vi "Manage Springboards.vi"() -> ()   [LabVIEW 2016]
panel:
  in  "Open in Explorer":bool
  in  "Open VI":bool
  in  "Delete":bool
  in  "Springboards List":i32[](listbox)
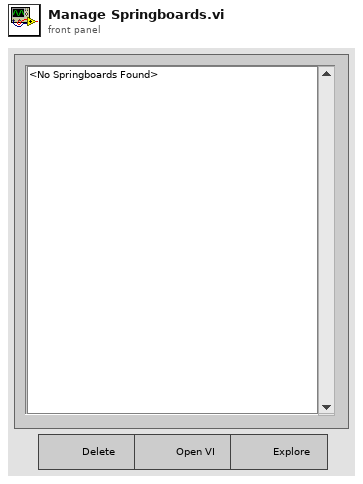
[diagram p1: front panel]
types:
  T1 = cluster{"Base Path":path, "Selected Items":i32[], "Springboard List":string[]}
  T2 = enum16{"Init", "Wait", "Delete", "Open", "Explore", "Exit"}
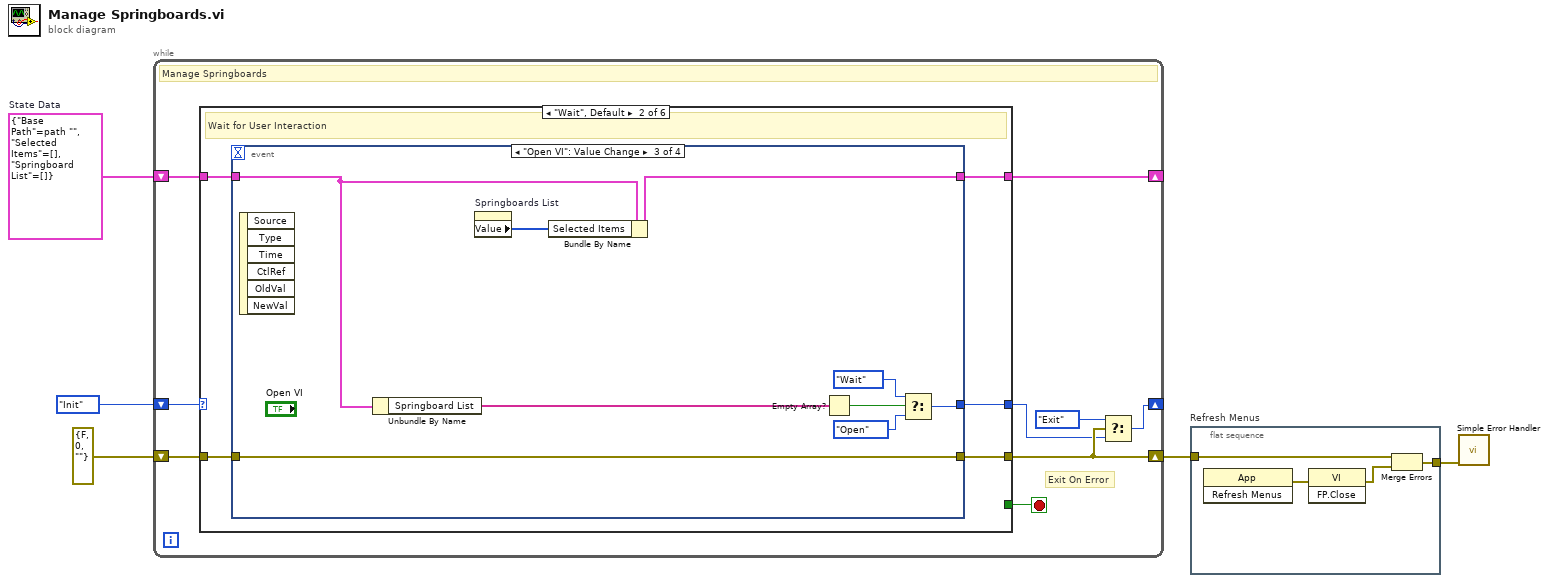
[diagram p0: block diagram]
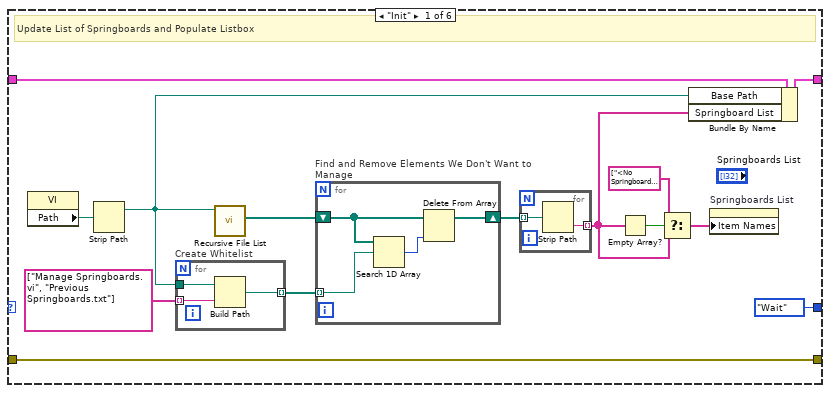
[diagram p2: hidden frame]
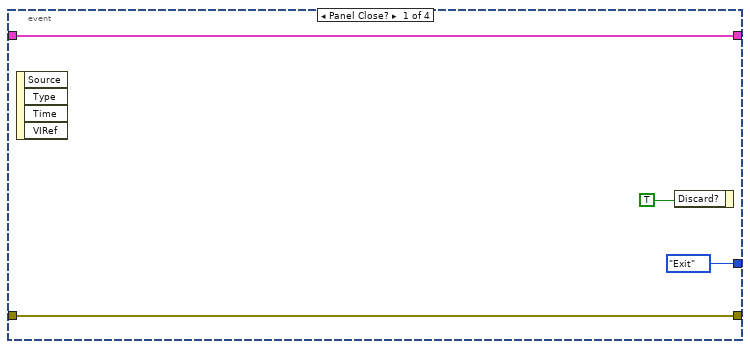
[diagram p3: hidden frame]
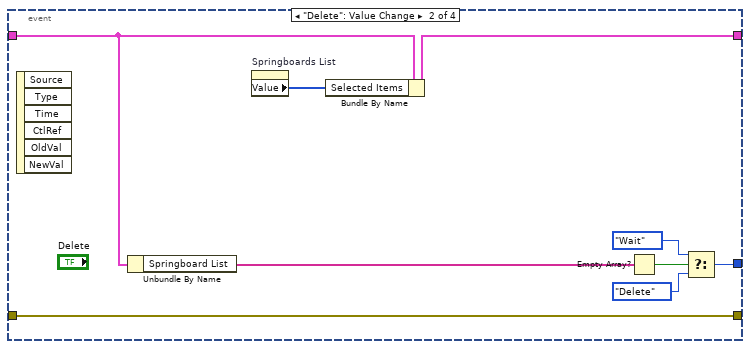
[diagram p4: hidden frame]
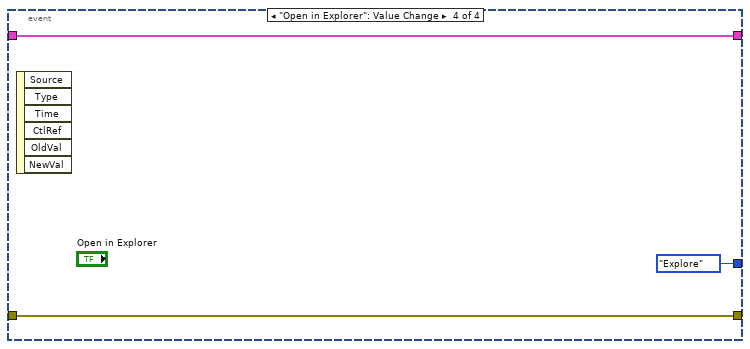
[diagram p5: hidden frame]
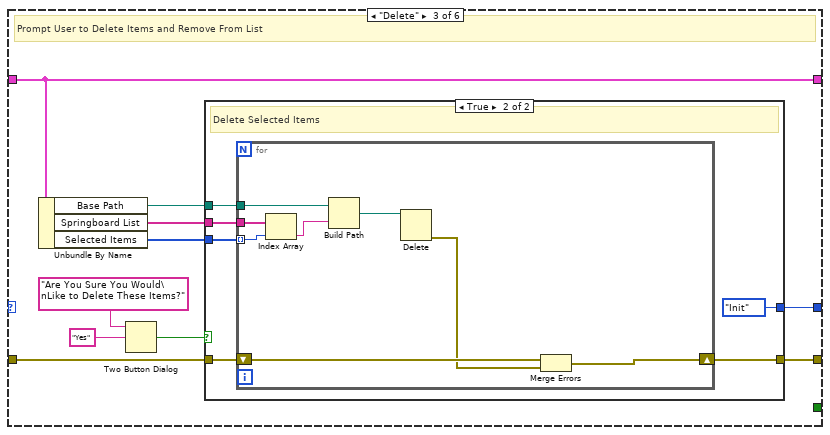
[diagram p6: hidden frame]
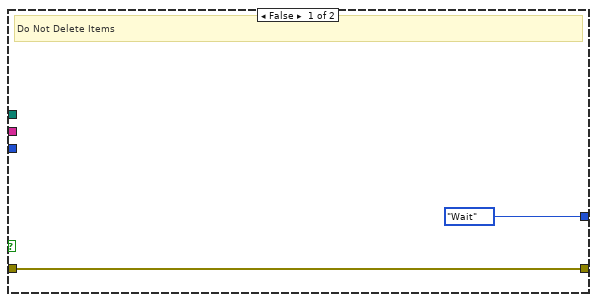
[diagram p7: hidden frame]
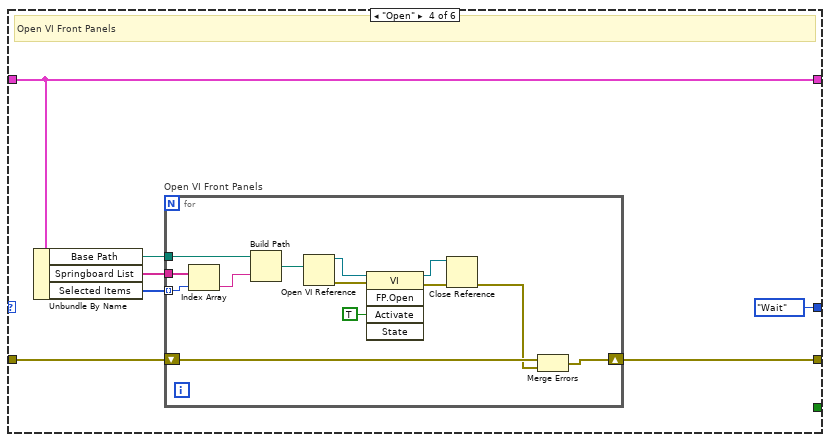
[diagram p8: hidden frame]
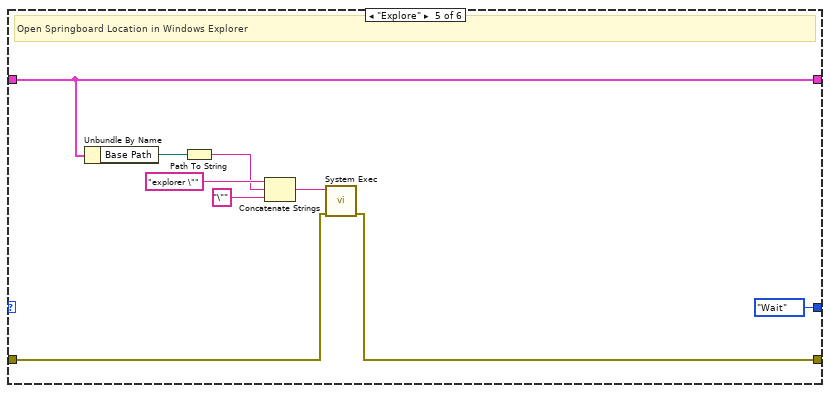
[diagram p9: hidden frame]
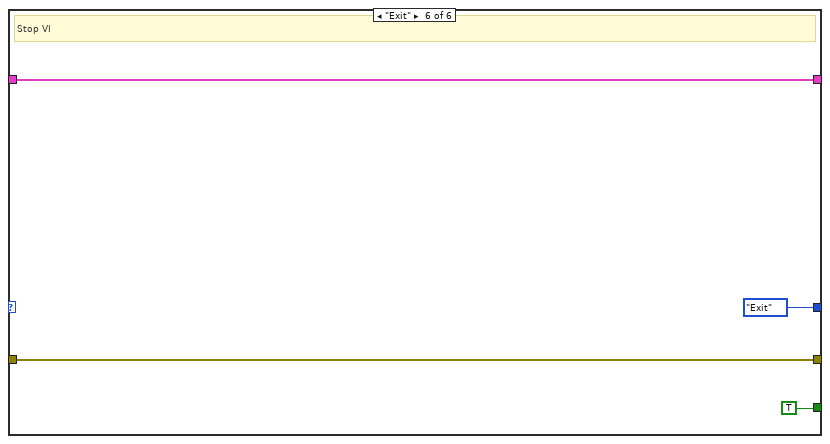
[diagram p10: hidden frame]
diagram:
  w3 = T1 {"Base Path"=path "", "Selected Items"=[], "Springboard List"=[]}  # State Data
  n1 = while {
    shift-right: [w9] -> _
    shift-left: T2."Init" -> [w13]
    shift-right: [w12] -> w2
    shift-left: errorcluster {"status"=FALSE, "code"=0, "source"=""} ("error constant") -> [w14]
    shift-right: [w7] -> _
    shift-left: w3 -> [w8]
    stop <- w6 stop-if-true
    # "Exit On Error"
    # "Manage Springboards"
    n2 = case shown="\"Wait\", Default" w13 {
      tunnel: w14 -> [w28 w42 w75 w95 w115 w126]
      tunnel: [w28 w41 w72 w94 w114 w126] -> w12
      tunnel: [T2."Wait" w40 w73 T2."Wait" T2."Wait" T2."Exit"] -> w11
      tunnel: w8 -> [w22 w39 w71 w99 w121 w124]
      tunnel: [w21 w38 w71 w99 w121 w124] -> w7
      tunnel: [_ _ _ _ _ TRUE] -> w6
      frame "Init" {
        # "Update List of Springboards and Populate Listbox"
        n3 = property class="VI"() -> ("Path"=w27:path)  [unwired: 2 in, 2 out]
        n4 = Strip Path(path=w27) -> (stripped path=w20:path)  [unwired: 1 out]
        n5 = for "Create Whitelist" {
          tunnel: w20 -> [w33]
          tunnel: [w32] -> w25 mode=indexing
          tunnel: string[] ["Manage Springboards.vi", "Previous Springboards.txt"] -> [w31] mode=indexing
          n6 = Build Path(base path=w33, name or relative path=w31) -> (appended path=w32:path)
        }
        n7 = call <vilib>:"Recursive File List.vi"("Folder Path"=w20) -> ("All Files in Dir"=w26:path[])  [unwired: 6 in, 4 out]
        n8 = for "Find and Remove Elements We Don't Want to Manage" {
          tunnel: w25 -> [w37] mode=indexing
          shift-right: [w35] -> w23
          shift-left: w26 -> [w36]
          n9 = Search 1D Array(1D array=w36, element=w37) -> (index of element=w34:i32)  [unwired: 1 in]
          n10 = Delete From Array(array=w36, index=w34) -> (array with subset deleted=w35:path[])  [unwired: 1 in, 1 out]
        }
        n11 = for {
          tunnel: w23 -> [w30] mode=indexing
          tunnel: [w29] -> w17 mode=indexing
          n12 = Strip Path(path=w30) -> (name=w29:string)  [unwired: 1 out]
        }
        n13 = Empty Array?(array=w17) -> (empty?=w18:bool)
        n14 = Select(t=string[] ["<No Springboards Found>"], s=w18, f=w17) -> (s? t:f=w15:string[])
        n15 = Bundle By Name(cluster=w22, "Base Path"=w20, "Springboard List"=w17) -> (w21:T1)
        n16 = property on="Springboards List" class="LstBox (strict)"("Item Names"=w15) -> ()  [unwired: 2 in, 2 out]
      }
      frame "Wait", Default {
        # "Wait for User Interaction"
        n17 = event shown="[2] \"Open VI\": Value Change" {
          selector: _ -> [_ _ _ _]
          dyn-events: _ -> [_ _ _ _]
          timeout: _ -> [_ _ _ _]
          tunnel: w42 -> [w46 w55 w64 w67]
          tunnel: [w46 w55 w64 w67] -> w41
          tunnel: [T2."Exit" w50 w58 T2."Explore"] -> w40
          tunnel: w39 -> [w43 w49 w57 w65]
          tunnel: [w43 w54 w63 w65] -> w38
          event Panel Close? {
            n18 = event-data() -> ()  [unwired: 1 in, 4 out]
            n19 = event-data("Discard?"=TRUE) -> ()  [unwired: 1 in, 1 out]
          }
          event "Delete": Value Change {
            n20 = event-data() -> ()  [unwired: 1 in, 6 out]
            n21 = Unbundle By Name(w49) -> ("Springboard List"=w48:string[])
            n22 = property on="Springboards List" class="LstBox (strict)"() -> ("Value"=w53:i32[])  [unwired: 2 in, 2 out]
            n23 = Bundle By Name(cluster=w49, "Selected Items"=w53) -> (w54:T1)
            n24 = Empty Array?(array=w48) -> (empty?=w47:bool)
            n25 = Select(t=T2."Wait", s=w47, f=T2."Delete") -> (s? t:f=w50:T2)
          }
          event "Open VI": Value Change {
            n26 = event-data() -> ()  [unwired: 1 in, 6 out]
            n27 = Unbundle By Name(w57) -> ("Springboard List"=w56:string[])
            n28 = property on="Springboards List" class="LstBox (strict)"() -> ("Value"=w62:i32[])  [unwired: 2 in, 2 out]
            n29 = Bundle By Name(cluster=w57, "Selected Items"=w62) -> (w63:T1)
            n30 = Empty Array?(array=w56) -> (empty?=w61:bool)
            n31 = Select(t=T2."Wait", s=w61, f=T2."Open") -> (s? t:f=w58:T2)
          }
          event "Open in Explorer": Value Change {
            n32 = event-data() -> ()  [unwired: 1 in, 6 out]
          }
        }
      }
      frame "Delete" {
        # "Prompt User to Delete Items and Remove From List"
        n33 = Unbundle By Name(w71) -> ("Base Path"=w70:path, "Springboard List"=w69:string[], "Selected Items"=w68:i32[])
        n34 = Two Button Dialog(message="Are You Sure You Would\nLike to Delete These Items?", 2:"Yes" ("T button name (\"OK\")")) -> (T button?=w74:bool)  [unwired: 1 in]
        n35 = case shown="True" w74 {
          tunnel: w75 -> [w78 w81]
          tunnel: [T2."Wait" T2."Init"] -> w73
          tunnel: [w78 w80] -> w72
          tunnel: w70 -> [_ w84]
          tunnel: w69 -> [_ w83]
          tunnel: w68 -> [_ w82]
          frame False {
            # "Do Not Delete Items"
          }
          frame True {
            # "Delete Selected Items"
            n36 = for {
              tunnel: w84 -> [w91]
              tunnel: w83 -> [w93]
              tunnel: w82 -> [w92] mode=indexing
              shift-right: [w88] -> w80
              shift-left: w81 -> [w87]
              n37 = Index Array(array=w93, index=w92) -> (element=w90:string)
              n38 = Build Path(base path=w91, name or relative path=w90) -> (appended path=w89:path)
              n39 = Delete(path (use dialog)=w89) -> (error out=w86:errorcluster)  [unwired: 4 in, 2 out]
              n40 = Merge Errors(w87, w86) -> (w88:errorcluster)
            }
          }
        }
      }
      frame "Open" {
        # "Open VI Front Panels"
        n41 = Unbundle By Name(w99) -> ("Base Path"=w96:path, "Springboard List"=w97:string[], "Selected Items"=w98:i32[])
        n42 = for "Open VI Front Panels" {
          tunnel: w98 -> [w112] mode=indexing
          tunnel: w97 -> [w113]
          tunnel: w96 -> [w111]
          shift-right: [w103] -> w94
          shift-left: w95 -> [w105]
          n43 = Index Array(array=w113, index=w112) -> (element=w110:string)
          n44 = Build Path(base path=w111, name or relative path=w110) -> (appended path=w109:path)
          n45 = Open VI Reference(vi path=w109) -> (vi reference=w107:refnum<vi>, error out=w108:errorcluster)  [unwired: 5 in]
          n46 = invoke class="VI" method="FP.Open"(reference=w107, error in=w108, "Activate"=TRUE ("Activate?")) -> (reference out=w101:refnum<vi>, error out=w104:errorcluster)  [unwired: 2 in, 3 out]
          n47 = Close Reference(reference=w101, error in (no error)=w104) -> (error out=w102:errorcluster)
          n48 = Merge Errors(w105, w102) -> (w103:errorcluster)
        }
      }
      frame "Explore" {
        # "Open Springboard Location in Windows Explorer"
        n49 = Unbundle By Name(w121) -> ("Base Path"=w120:path)
        n50 = Path To String(path=w120) -> (string=w117:string)
        n51 = Concatenate Strings("explorer \"" ("string"), w117, "\"" ("string")) -> (w116:string)
        n52 = call <vilib>:"System Exec.vi"("error in (no error)"=w115, "command line"=w116) -> ("error out"=w114:errorcluster)  [unwired: 6 in, 3 out]
      }
      frame "Exit" {
        # "Stop VI"
      }
    }
    n53 = Select(t=T2."Exit", s=w12, f=w11) -> (s? t:f=w9:T2)
  }
  n54 = flat-sequence "Refresh Menus" {
    tunnel: w2 -> [w130]
    tunnel: [w129] -> w1
    frame #0 {
      n55 = invoke class="App" method="Refresh Menus"() -> (error out=w128:errorcluster)  [unwired: 3 in, 2 out]
      n56 = invoke class="VI" method="FP.Close"(error in=w128) -> (error out=w127:errorcluster)  [unwired: 2 in, 2 out]
      n57 = Merge Errors(w130, w127) -> (w129:errorcluster)
    }
  }
  n58 = call <vilib>:"Simple Error Handler.vi"("error in (no error)"=w1) -> ()  [unwired: 4 in, 5 out]
